vi "Sensors signals.vi"(11 "error in (no error)":errorcluster) -> ()   [LabVIEW 2019]
uses:
  <vilib>/Platform/TimedLoop/XDataNode/timing_clust.ctl
  <vilib>/Platform/TimedLoop/XDataNode/nitl_modes.ctl
  <vilib>/Platform/TimedLoop/XDataNode/wakeup.ctl
  Global.vi
  <vilib>/Utility/error.llb/Error Cluster From Error Code.vi
  <vilib>/myRIO/Common/Instrument Driver Framework/myRIO v1.0/AI/vis/myRIO v1.0 Read AI.vi
  <vilib>/platform/TimedLoop/XDataNode/XDataNode.xnode
  <vilib>/myRIO/Instrument Drivers/Onboard IO/AI/AI.lvlib
  <vilib>/Platform/TimedLoop/XDataNode/XDNodeRunTimeDep.lvlib
  <vilib>/Analysis/NI_AAL_SigProc.lvlib
  <vilib>/ptbypt/NI_PtbyPt.lvlib
panel:
  in  "Tab Control 2":enum32{"Graph", "Filter controls"}(tab)
  out "Sensors data":T1(graph)
  in  "Sensor Tare":bool
  in  "Tare sensor 2":dbl
  in  "Tare sensor 1":dbl
  in  "Width":i32(slide)=10 scale=0.0..500.0
  in  "Threshold":dbl(slide)=4.897959183673464 scale=-60.0..60.0
  out "Locations":dbl[](array[numeric])
  out "element":dbl
  out "size(s)":i32
  in  "Ts":dbl=0.002
  in  "Tf":dbl=0.01 format="%#_13g"
  in  "Tf 2":dbl=1e-05
  in  "Ts 2":dbl=3e-08
  in  "sample length":i32=30
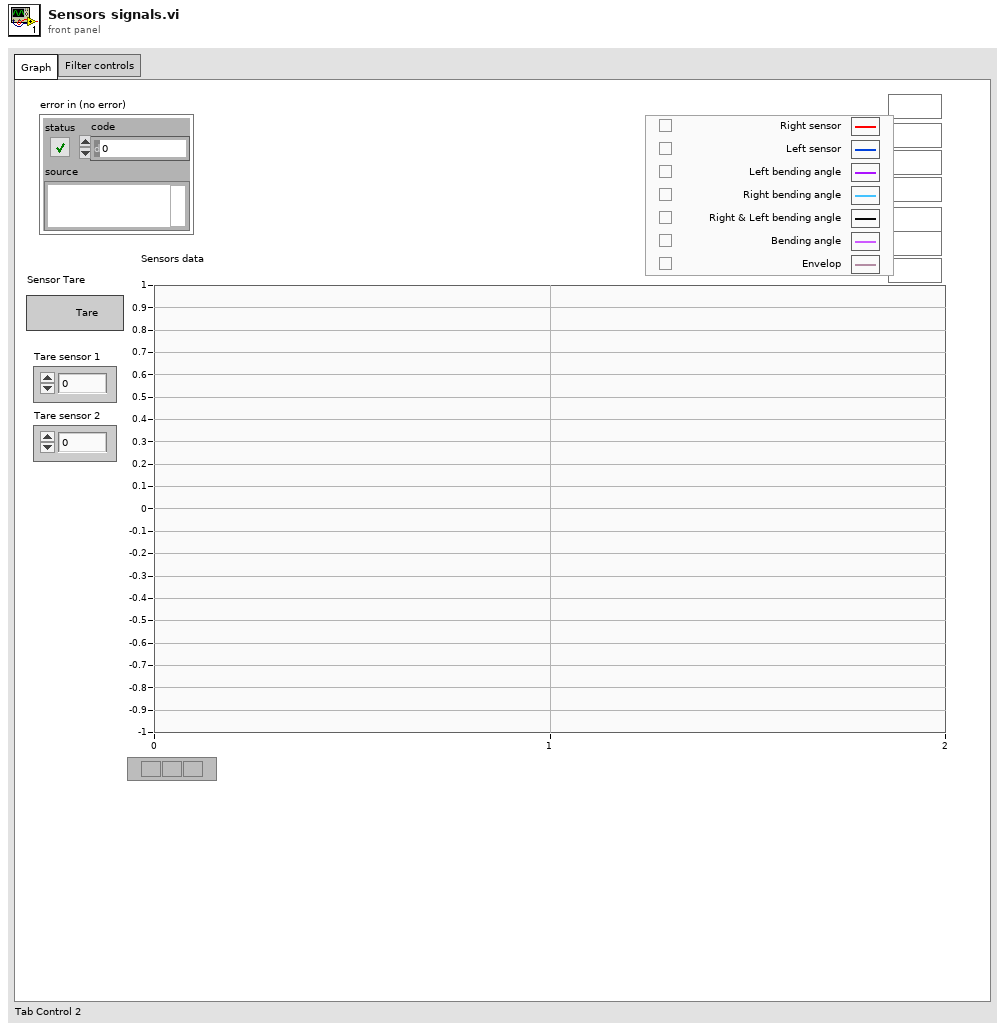
[diagram p1: front panel]
types:
  T1 = cluster{"yf1":dbl, "yf2":dbl, dbl, "Right bending angle":dbl, dbl, dbl, dbl}
  T2 = cluster{"yf1":dbl, "yf2":dbl, "Left bending angle":dbl, "Right bending angle":dbl, dbl, dbl, dbl}[]
  T3 = typedef "XDNodeRunTimeDep.lvlib/timing_clust.ctl" = cluster{"Expected End [f-1]":u64, "Actual End [f-1]":u64, "Finished Late? [f-1]":bool, "Expected End [i-1]":u64, "Actual End [i-1]":u64, "Finished Late? [i-1]":bool, "Expected Start [i]":u64, "Actual Start [i]":u64, "Expected Start [f]":u64, "Actual Start [f]":u64, "Source Name":string, "Structure Name":string, "Period":i64, "Deadline":i64, "Offset":i64, "Start":i64, "Priority":i32, "Timeout":i32, "Mode":T4, "Wakeup Reason":T5, "Error":errorcluster, "Source Type":string, "Secondary Source Type":string, "Global End Time":u64, "Global Start Time":u64, "Frame Duration":u64, "Iteration Duration":u64, "Assigned CPU":i32, "I/O Scan Engine Mode":u32}
  T4 = typedef "XDNodeRunTimeDep.lvlib/nitl_modes.ctl" = enum32{"No Change", "Process missed periods, maintain original phase", "Discard missed periods, maintain original phase", "Process missed periods, ignore original phase", "Discard missed periods, ignore original phase"}
  T5 = typedef "XDNodeRunTimeDep.lvlib/wakeup.ctl" = enum32{"Normal", "Aborted", "Asynchronous wakeup", "Timing source error", "Timed loop error", "Timeout"}
  T6 = typedef "AI.lvlib/AI Reference.ctl" = cluster{"myRIO Reference":T7, "AI Channels List":T11, "AI Scaling Constants List":T13}
  T7 = typedef "myRIO Generic Hardware Reference.ctl" = cluster{"myRIO Model":T8, "myRIO Hardware Reference":T9}
  T8 = typedef "Hardware Version Enum.ctl" = enum16{"Unknown", "myRIO-1900", "myRIO-1950", "roboRIO", "NI ELVIS RIO CM", "ELVIS III"}
  T9 = typedef "myRIO v1.0 Reference.ctl" = cluster{"Generic FPGA Reference":T10, "Allow multiple opens":bool}
  T10 = typedef "Generic FPGA Reference.ctl" = refnum<k20>
  T11 = typedef "AI Channels List.ctl" = T12[]
  T12 = typedef "AI Channels Enum.ctl" = enum16{"Not Connected", "AudioIn/Left", "AudioIn/Right", "C/AI0", "C/AI1", "A/AI0", "A/AI1", "A/AI2", "A/AI3", "A/AI4", "A/AI5", "A/AI6", "A/AI7", "B/AI0", "B/AI1", "B/AI2", "B/AI3", "B/AI4", "B/AI5", "B/AI6", "B/AI7", "AI/AI0", "AI/AI1", "AI/AI2", "AI/AI3", "A/AI0 (DIFF)", "A/AI1 (DIFF)", "A/AI2 (DIFF)", "A/AI3 (DIFF)", "B/AI0 (DIFF)", "B/AI1 (DIFF)", "B/AI2 (DIFF)", "B/AI3 (DIFF)"}
  T13 = typedef "Analog Scaling Constants List.ctl" = T14[]
  T14 = typedef "Analog Scaling Constants.ctl" = cluster{"LSB Weight (Volts)":dbl, "Offset (Volts)":dbl, "Signed?":bool}
  T15 = cluster{"Left bending angle":dbl, "Right bending angle":dbl}
  T16 = cluster{"yf1":dbl, "yf2":dbl, "Left bending angle":dbl, "Right bending angle":dbl, dbl, dbl, "mean":dbl}
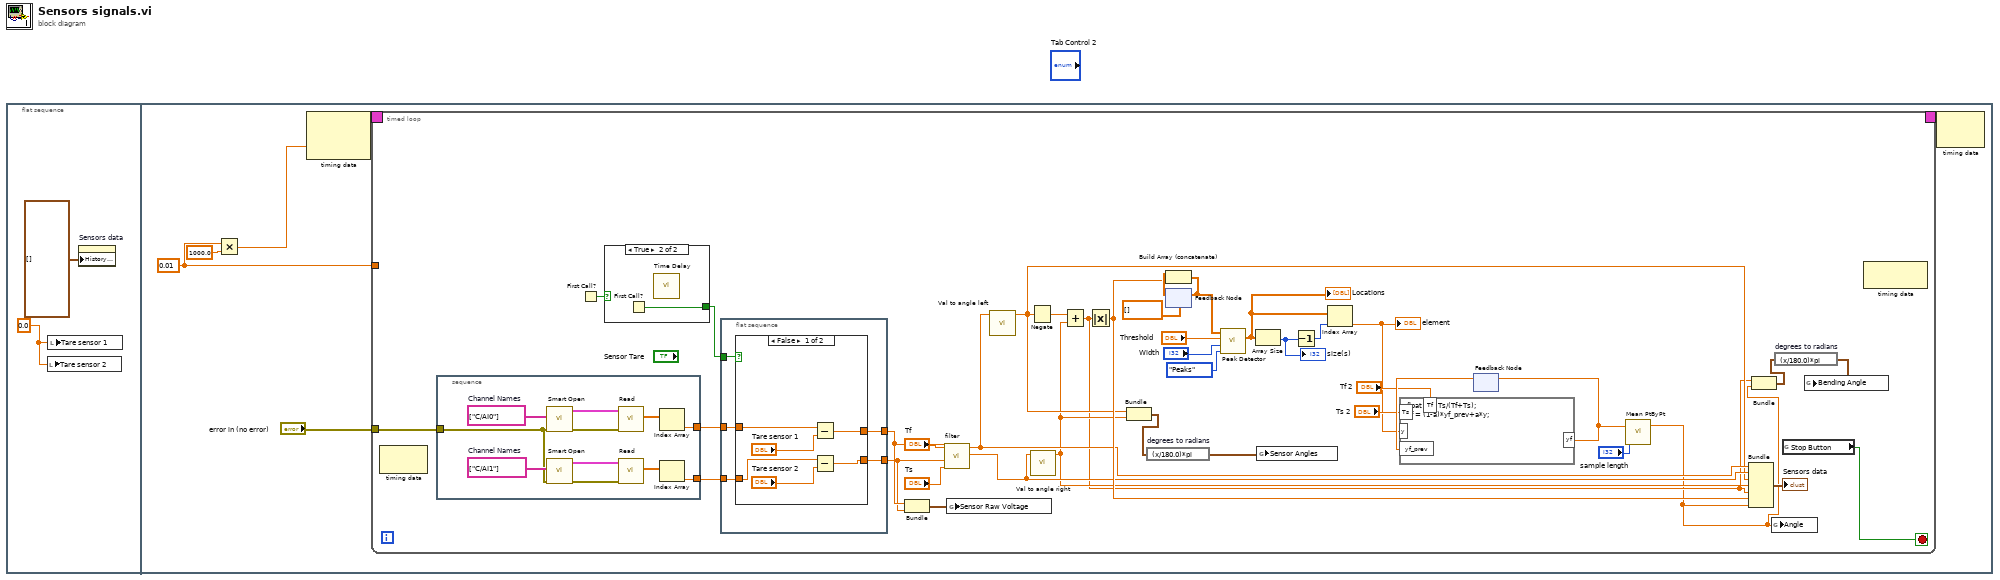
[diagram p0: block diagram]
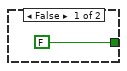
[diagram p2: hidden frame]
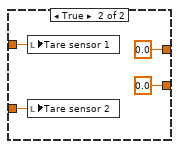
[diagram p3: hidden frame]
diagram:
  n1 = flat-sequence {
    frame #0 {
      w1 = 0.0 ("Tare sensor 1")
      n2 = local write "Tare sensor 2"(w1) -> ()
      n3 = local write "Tare sensor 1"(w1) -> ()
      n4 = property on="Sensors data" class="WFChart (strict)"("History Data"=T2 []) -> ()  [unwired: 2 in, 2 out]
    }
    frame #1 {
      w3 = 0.01
      n5 = Multiply(x=w3, y=1000.0) -> (x*y=w4:dbl)
      n6 = node-c288(w4) -> (w8:T3)  [unwired: 1 in]
      n7 = timed-loop {
        tunnel: "error in (no error)" -> [w42]
        timing: w8 -> [_]
        timing-out: [_] -> w7
        tunnel: w3 -> [_]
        stop <- w43 stop-if-true
        n8 = node-c288() -> ()  [unwired: 1 in, 1 out]
        n9 = stacked-sequence {
          tunnel: [w75] -> w46
          tunnel: [w69] -> w47
          tunnel: w42 -> [w67]
          frame #0 {
            w70 = tag[] ["C/AI0"]  # Channel Names
            w74 = tag[] ["C/AI1"]  # Channel Names
            n10 = call <vilib>:"Smart Open.vi"("error in (no error)"=w67, "Channel Names"=w70) -> ("error out"=w73:errorcluster, "AI Ref Out"=w72:T6)  [unwired: 8 in]
            n11 = call <vilib>:"Smart Open.vi"("error in (no error)"=w67, "Channel Names"=w74) -> ("error out"=w77:errorcluster, "AI Ref Out"=w76:T6)  [unwired: 8 in]
            n12 = call <vilib>:"Read.vi"("error in (no error)"=w73, "AI Ref In"=w72) -> ("Values"=w71:dbl[])  [unwired: 7 in, 2 out]
            n13 = call <vilib>:"Read.vi"("error in (no error)"=w77, "AI Ref In"=w76) -> ("Values"=w68:dbl[])  [unwired: 7 in, 2 out]
            n14 = Index Array(array=w71) -> (element=w69:dbl)  [unwired: 1 in]
            n15 = Index Array(array=w68) -> (element=w75:dbl)  [unwired: 1 in]
          }
        }
        n16 = First Call?() -> (First Call?: T/F=w22:bool)
        n17 = case shown="True" w22 {
          tunnel: [FALSE ("initialize: T/F") w49] -> w19
          frame False {
          }
          frame True {
            n18 = First Call?() -> (First Call?: T/F=w49:bool)
            n19 = call "Time Delay"() -> ()  [unwired: 11 in, 1 out]
          }
        }
        n20 = flat-sequence {
          tunnel: [w56] -> w21
          tunnel: [w55] -> w20
          tunnel: w47 -> [w54]
          tunnel: w46 -> [w53]
          tunnel: w19 -> [w52]
          frame #0 {
            n21 = case shown="False" w52 {
              tunnel: [w62 0.0] -> w55
              tunnel: [w61 0.0] -> w56
              tunnel: w54 -> [w60 w64]
              tunnel: w53 -> [w59 w63]
              frame False {
                n22 = Subtract(x=w60, y="Tare sensor 1") -> (x-y=w61:dbl)
                n23 = Subtract(x=w59, y="Tare sensor 2") -> (x-y=w62:dbl)
              }
              frame True {
                n24 = local write "Tare sensor 1"(w64) -> ()
                n25 = local write "Tare sensor 2"(w63) -> ()
              }
            }
          }
        }
        n26 = Bundle(w21, w20) -> (w44:cluster{dbl, dbl})  [unwired: 1 in]
        n27 = call "filter.vi"("Ts"="Ts", "y2"=w20, "y1"=w21, "Tf"="Tf") -> ("yf2"=w17:dbl, "yf1"=w18:dbl)  [unwired: 6 in]
        n28 = global write "Global.vi" "Sensor Raw Voltage"(w44) -> ()
        n29 = call "Val to angle left.vi"("Sensor val"=w18) -> ("Left bending angle"=w16:dbl)  [unwired: 10 in]
        n30 = Negate(x=w16) -> (-x=w45:dbl)
        n31 = call "Val to angle right.vi"("Sensor val"=w17) -> ("Right bending angle"=w15:dbl)  [unwired: 10 in]
        n32 = Add(x=w45, y=w15) -> (x+y=w14:dbl)
        n33 = Absolute Value(x=w14) -> (abs(x)=w24:dbl)
        n34 = Bundle("Left bending angle"=w16, "Right bending angle"=w15) -> (w12:T15)  [unwired: 1 in]
        n35 = expression code="(x/180.0)*pi" "degrees to radians"(w12) -> (w11:T15)
        n36 = feedback #1(dbl[] []) -> (w39:dbl[])
        n37 = Build Array (concatenate)(w39, w24) -> (w34:dbl[])
        n38 = feedback-in #1(w34) -> ()
        n39 = call <vilib>:"Peak Detector.vi"("peaks/valleys"=enum32{"Peaks", "Valleys"}."Peaks", "width"="Width", "threshold"="Threshold", "X"=w34) -> ("Amplitudes"=w27:dbl[])  [unwired: 3 in, 4 out]
        "Locations" <- w27
        n40 = Array Size(array=w27) -> (size(s)=w32:i32)
        "size(s)" <- w32
        n41 = global write "Global.vi" "Sensor Angles"(w11) -> ()
        n42 = Decrement(x=w32) -> (x-1=w33:i32)
        n43 = Index Array(array=w27, index=w33) -> (element=w26:dbl)
        "element" <- w26
        n44 = feedback #2() -> (w31:dbl)  [unwired: 1 in]
        n45 = formula code="float a = Ts/(Tf+Ts);\nyf = (1-a)*yf_prev+a*y;"("Tf"="Tf 2", "Ts"="Ts 2", "y"=w26, "yf_prev"=w31) -> ("yf"=w25:dbl)
        n46 = feedback-in #2(w25) -> ()
        n47 = call <vilib>:"Mean PtByPt.vi"("x"=w25, "sample length"="sample length") -> ("mean"=w13:dbl)  [unwired: 2 in, 1 out]
        n48 = Bundle("yf1"=w18, "yf2"=w17, "Left bending angle"=w16, "Right bending angle"=w15, w14, w24, "mean"=w13) -> (→"Sensors data":T16)  [unwired: 1 in]
        n49 = Bundle(w14, "mean"=w13) -> (w10:cluster{dbl, "mean":dbl})  [unwired: 1 in]
        n50 = global write "Global.vi" "Angle"(w13) -> ()
        n51 = expression code="(x/180.0)*pi" "degrees to radians"(w10) -> (w9:cluster{dbl, "mean":dbl})
        n52 = global read "Global.vi" "Stop Button"() -> (w43:bool)
        n53 = global write "Global.vi" "Bending Angle"(w9) -> ()
        n54 = node-c288() -> ()  [unwired: 1 in, 1 out]
      }
      n55 = node-c288(w7) -> ()  [unwired: 1 out]
    }
  }
